vi "Exclusive Or.vi"(0 "String":string="\tB01F") -> (4 "String OutPut":string, 6 "HEX String OutPut":string, 8 "Exclusive Or":u8[](array[numeric]) format="%.0x")   [LabVIEW 2020, in "UART.lvlib"]
uses:
  UART/UART.lvlib
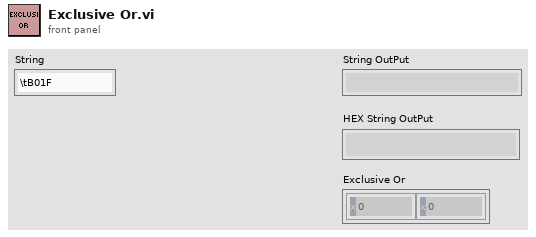
[diagram p1: front panel]
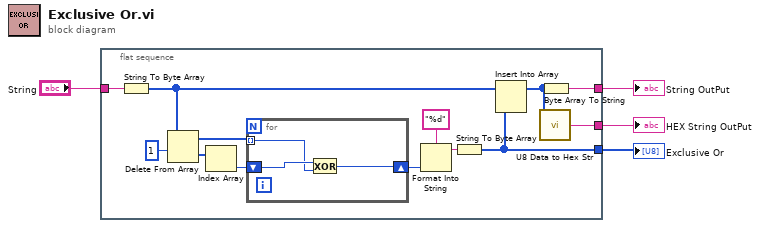
[diagram p0: block diagram]
diagram:
  n1 = flat-sequence {
    tunnel: "String" -> [w13]
    tunnel: [w8] -> w3
    tunnel: [w7] -> w2
    tunnel: [w6] -> w1
    frame #0 {
      n2 = String To Byte Array(string=w13) -> (unsigned byte array=w9:u8[])
      n3 = Delete From Array(array=w9, length=1) -> (deleted portion=w15:u8[], array with subset deleted=w16:u8[])  [unwired: 1 in]
      n4 = Index Array(array=w15) -> (element=w14:u8)  [unwired: 1 in]
      n5 = for {
        tunnel: w16 -> [w18] mode=indexing
        shift-right: [w20] -> w12
        shift-left: w14 -> [w19]
        n6 = Exclusive Or(1:w18, 2:w19) -> (0:w20:u8)
      }
      n7 = Format Into String(format string="%d", w12) -> (resulting string=w10:string)  [unwired: 2 in, 1 out]
      n8 = String To Byte Array(string=w10) -> (unsigned byte array=w7:u8[])
      n9 = Insert Into Array(array=w9, new element=w7) -> (w5:u8[])  [unwired: 1 in]
      n10 = call "U8 Data to Hex Str.vi"("u8 Data[]"=w5) -> ("HEX String (0-9,A-F)"=w6:string)
      n11 = Byte Array To String(unsigned byte array=w5) -> (string=w8:string)
    }
  }
  "String OutPut" <- w3
  "Exclusive Or" <- w2
  "HEX String OutPut" <- w1
